vi "RoutineControl.vi"(5 "LogSuspend":bool, 8 "error in":errorcluster, 10 "HexStirngArray":string, 11 "UdsHandleIn":T2={"LogPath"=path "", "LogEnabled"=FALSE, "isOpen"=FALSE, "LogContent"="", "Adapter"="CAN0", "MCanHandle"={"MCanAdapter"=refnum}, "TransmittId"=0, "ReceiveId"=0}) -> (0 "error out":errorcluster, 2 "Response":string, 3 "UdsHandleOut":T2={"LogPath"=path "", "LogEnabled"=FALSE, "isOpen"=FALSE, "LogContent"="", "Adapter"="CAN0", "MCanHandle"={"MCanAdapter"=refnum}, "TransmittId"=0, "ReceiveId"=0})   [LabVIEW 2011, in "Konvolucio MUDS150628.lvlib"]
uses:
  <instrlib>/Konvolucio MUDS150628/Konvolucio MUDS150628.lvlib
  <instrlib>/Konvolucio MUDS150628/Types/UdsHandleType.ctl
  <instrlib>/Konvolucio MCAN120803/Types/MCanHandleType.ctl
  C:/Program Files/National Instruments/LabVIEW 2011/instr.lib/Konvolucio MCAN120803/Private/Konvolucio.MCAN120803.dll
  Konvolucio MCAN120803/Private/Konvolucio.MCAN120803.dll
  <instrlib>/Konvolucio MCAN120803/Konvolucio MCAN120803.lvlib
panel:
  in  "Subfunction":T1(ring)=enum."RequestRoutineResults"
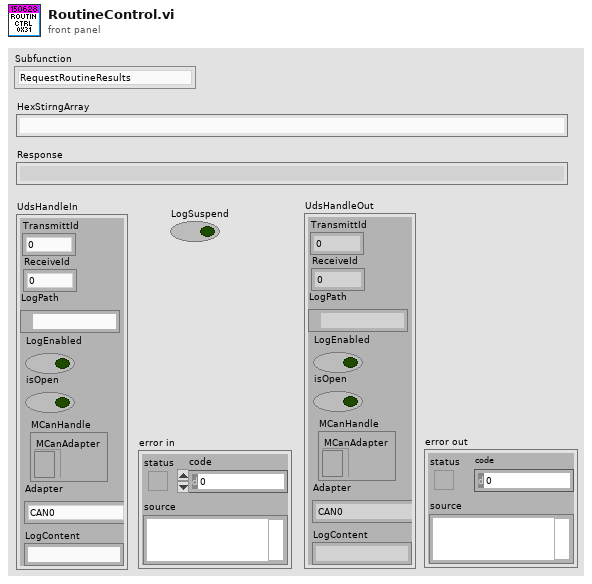
[diagram p1: front panel]
types:
  T1 = enum16{"StartRoutnie", "StopRoutine", "RequestRoutineResults"}
  T2 = typedef "Konvolucio MUDS150628.lvlib/UdsHandleType.ctl" = cluster{"LogPath":path, "LogEnabled":bool, "isOpen":bool, "LogContent":string, "Adapter":string, "MCanHandle":T3, "TransmittId":u32, "ReceiveId":u32}
  T3 = typedef "Konvolucio MCAN120803.lvlib/MCanHandleType.ctl" = cluster{"MCanAdapter":refnum<k24>}
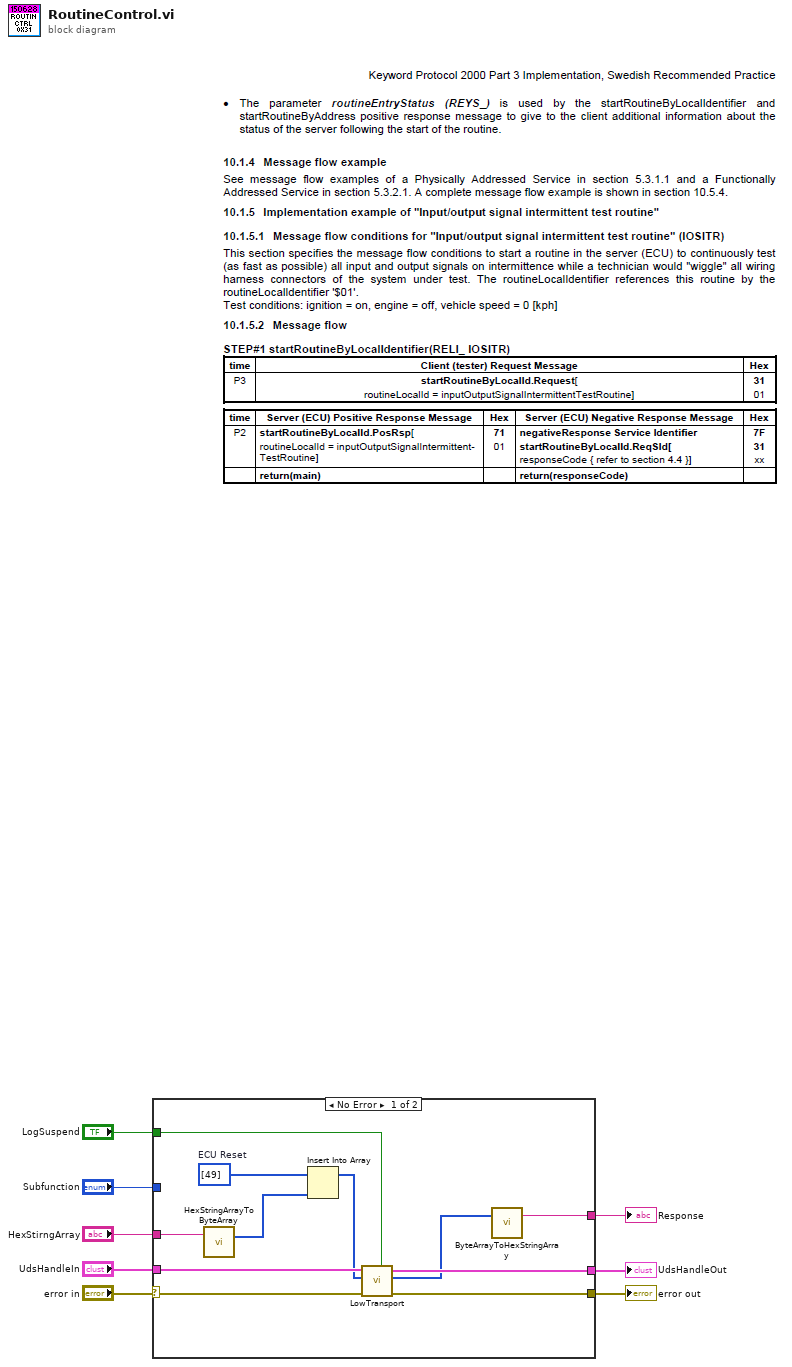
[diagram p0: block diagram]
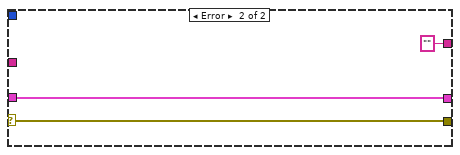
[diagram p2: hidden frame]
diagram:
  n1 = case shown="No Error" "error in" {
    selector: "error in" -> [w18 w22]
    tunnel: "UdsHandleIn" -> [w19 w21]
    tunnel: [w17 w22] -> w6
    tunnel: [w16 w21] -> w5
    tunnel: "LogSuspend" -> [w15 _]
    tunnel: "Subfunction" -> [_ _]
    tunnel: [w11 "" ("HexStringArrayOut")] -> w2
    tunnel: "HexStirngArray" -> [w9 _]
    frame No Error {
      w14 = u8[] [49]  # ECU Reset
      n2 = call <instrlib>:"HexStringArrayToByteArray.vi"("HexStirngArray"=w9) -> ("ByteArrayOut"=w10:u8[])  [unwired: 2 in]
      n3 = Insert Into Array(array=w14, new element=w10) -> (w13:u8[])  [unwired: 1 in]
      n4 = call <instrlib>:"LowTransport.vi"("LogSuspend"=w15, "error in"=w18, "Request"=w13, "HandleIn"=w19) -> ("error out"=w17:errorcluster, "Response"=w12:u8[], "HandleOut"=w16:T2)  [unwired: 5 in]
      n5 = call <instrlib>:"ByteArrayToHexStringArray.vi"("ByteArrayIn"=w12) -> ("HexStringArrayOut"=w11:string)  [unwired: 2 in]
    }
    frame Error {
    }
  }
  "error out" <- w6
  "UdsHandleOut" <- w5
  "Response" <- w2
